vi "AlliGator Check Invalid Python Plugin Input Parameter Types.vi"(8 "error in (no error)":errorcluster, 9 "Source":string, 11 "Invalid Parameter Types":string[](array[string])) -> (0 "error out":errorcluster)   [LabVIEW 2021, in "AlliGator Python Plugins.lvlib"]
doc: "Formats error with invalid input parameter message."
uses:
  AlliGator Python Plugins.lvlib
  <vilib>/Utility/error.llb/Error Cluster From Error Code.vi
  <vilib>/ErrorRing/Error Ring.xnode
  Strings/Strings.lvlib
panel:
  # "see the AlliGator License on the block diagram (Ctrl+E or Window:Show Block Diagram)"
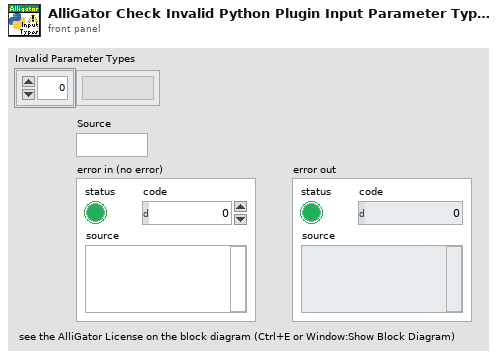
[diagram p1: front panel]
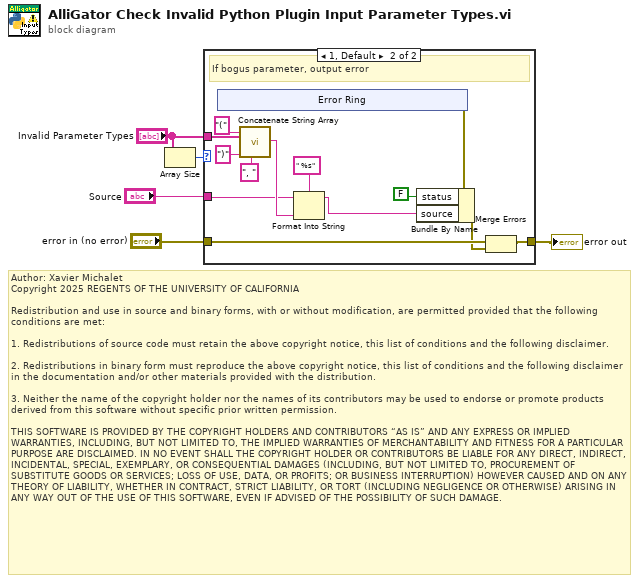
[diagram p0: block diagram]
diagram:
  # "Author: Xavier Michalet\nCopyright 2025 REGENTS OF THE UNIVERSITY OF CALIFORNIA\n\nRedistribution and use in source and binary forms, with or without modification, are permitted provided that the following conditions are met:\n\n1. Redistributions of source code must retain the above copyright notice, this list of conditions and the following disclaimer.\n\n2. Redistributions in binary form must reproduce the above copyright notice, this list of conditions and the following disclaimer in the documentation and/or other materials provided with the distribution.\n\n3. Neither the name of the copyright holder nor the names of its contributors may be used to endorse or promote products derived from this software without specific prior written permission.\n\nTHIS SOFTWARE IS PROVIDED BY THE COPYRIGHT HOLDERS AND CONTRIBUTORS “AS IS” AND ANY EXPRESS OR IMPLIED WARRANTIES, INCLUDING, BUT NOT LIMITED TO, THE IMPLIED WARRANTIES OF MERCHANTABILITY AND FITNESS FOR A PARTICULAR PURPOSE ARE DISCLAIMED. IN NO EVENT SHALL THE COPYRIGHT HOLDER OR CONTRIBUTORS BE LIABLE FOR ANY DIRECT, INDIRECT, INCIDENTAL, SPECIAL, EXEMPLARY, OR CONSEQUENTIAL DAMAGES (INCLUDING, BUT NOT LIMITED TO, PROCUREMENT OF SUBSTITUTE GOODS OR SERVICES; LOSS OF USE, DATA, OR PROFITS; OR BUSINESS INTERRUPTION) HOWEVER CAUSED AND ON ANY THEORY OF LIABILITY, WHETHER IN CONTRACT, STRICT LIABILITY, OR TORT (INCLUDING NEGLIGENCE OR OTHERWISE) ARISING IN ANY WAY OUT OF THE USE OF THIS SOFTWARE, EVEN IF ADVISED OF THE POSSIBILITY OF SUCH DAMAGE."
  n1 = Array Size(array="Invalid Parameter Types") -> (size(s)=w3:i32)
  n2 = case shown="1, Default" w3 {
    tunnel: "Invalid Parameter Types" -> [_ w19]
    tunnel: "error in (no error)" -> [w6 w16]
    tunnel: [w6 w17] -> w5
    tunnel: "Source" -> [_ w11]
    frame 0 {
    }
    frame 1, Default {
      # "If bogus parameter, output error"
      n3 = xnode "Error Ring"() -> ("error out"=w8:errorcluster)
      n4 = call "Concatenate String Array.vi"("Separator (TAB)"=", ", "Suffix (\"\")"=")" ("Suffix (\"\")"), "String Array"=w19, "Prefix (\"\")"="(" ("Prefix (\"\")")) -> ("Formatted String"=w15:string)  [unwired: 7 in]
      n5 = Format Into String(format string=" %s", initial string=w11, w15) -> (resulting string=w9:string)  [unwired: 1 in, 1 out]
      n6 = Bundle By Name(cluster=w8, "status"=FALSE, "source"=w9) -> (w7:errorcluster)
      n7 = Merge Errors(w16, w7) -> (w17:errorcluster)
    }
  }
  "error out" <- w5
